vi "Toggle Lift Ears.vi"(8 "Delay":dbl, 9 "Distance Threshold":dbl, 10 "Avg Distance":dbl, 11 "Robot Mode":T1=enum."Teleop Enabled") -> (3 "Lift Output":bool)   [LabVIEW 2013]
uses:
  <vilib>/Rock Robotics/WPI/DriverStation/WPI_DriverStationRobotMode2.ctl
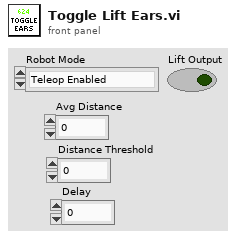
[diagram p1: front panel]
types:
  T1 = typedef "WPI_DriverStationRobotMode2.ctl" = enum16{"Autonomous Disabled", "Autonomous Enabled", "Teleop Disabled", "Teleop Enabled", "Timeout", "Finish", "Test Disabled", "Test Enabled"}
  T2 = enum16{"Wait for Auton", "Wait for Encoders", "On"}
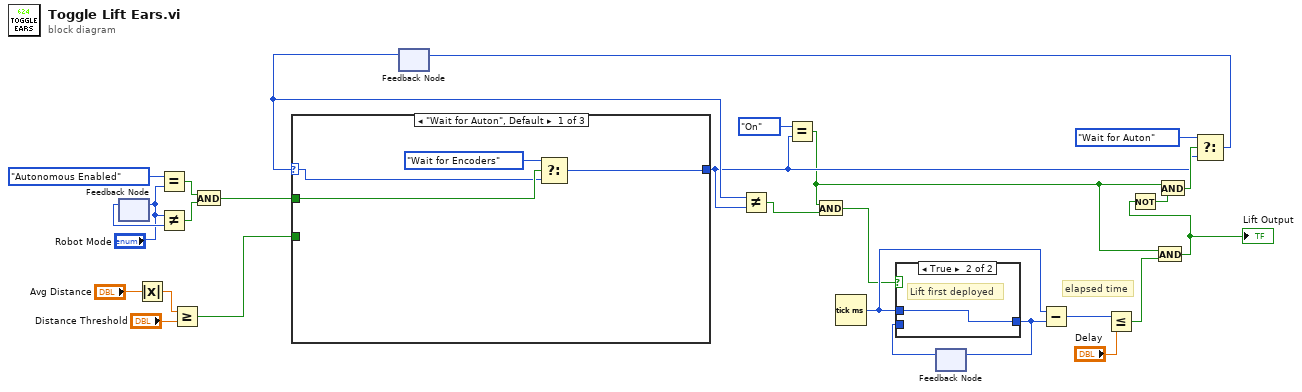
[diagram p0: block diagram]
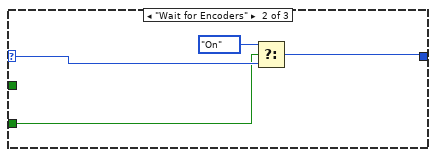
[diagram p3: hidden frame]
diagram:
  # "elapsed time"
  n1 = feedback #1() -> (w24:T1)  [unwired: 1 in]
  n2 = feedback-in #1("Robot Mode") -> ()
  n3 = Absolute Value(x="Avg Distance") -> (abs(x)=w17:dbl)
  n4 = Equal?(x=WPI_DriverStationRobotMode2."Autonomous Enabled", y="Robot Mode") -> (x = y?=w26:bool)
  n5 = Not Equal?(x="Robot Mode", y=w24) -> (x != y?=w27:bool)
  n6 = Greater Or Equal?(x=w17, y="Distance Threshold") -> (x >= y?=w21:bool)
  n7 = And(x=w26, y=w27) -> (x .and. y?=w22:bool)
  n8 = feedback #2() -> (w7:T2)  [unwired: 1 in]
  n9 = case shown="\"Wait for Auton\", Default" w7 {
    selector: w7 -> [w30 w34 w36]
    tunnel: w22 -> [w31 _ _]
    tunnel: [w28 w33 w36] -> w6
    tunnel: w21 -> [_ w32 _]
    frame "Wait for Auton", Default {
      n10 = Select(t=T2."Wait for Encoders", s=w31, f=w30) -> (s? t:f=w28:T2)
    }
    frame "Wait for Encoders" {
      n11 = Select(t=T2."On", s=w32, f=w34) -> (s? t:f=w33:T2)
    }
    frame "On" {
    }
  }
  n12 = Not Equal?(x=w7, y=w6) -> (x != y?=w5:bool)
  n13 = Equal?(x=T2."On" ("y"), y=w6) -> (x = y?=w3:bool)
  n14 = And(x=w3, y=w5) -> (x .and. y?=w4:bool)
  n15 = Tick Count (ms)() -> (millisecond timer value=w12:u32)
  n16 = feedback #3() -> (w14:u32)  [unwired: 1 in]
  n17 = case shown="True" w4 {
    tunnel: w14 -> [w37 _]
    tunnel: [w37 w38] -> w13
    tunnel: w12 -> [_ w38]
    frame False {
    }
    frame True {
      # "Lift first deployed"
    }
  }
  n18 = feedback-in #3(w13) -> ()
  n19 = Subtract(x=w12, y=w13) -> (x-y=w15:u32)
  n20 = Less Or Equal?(x=w15, y="Delay") -> (x <= y?=w2:bool)
  n21 = And(x=w3, y=w2) -> (x .and. y?=w1:bool)
  "Lift Output" <- w1
  n22 = Not(x=w1) -> (.not. x?=w10:bool)
  n23 = And(x=w3, y=w10) -> (x .and. y?=w9:bool)
  n24 = Select(t=T2."Wait for Auton", s=w9, f=w6) -> (s? t:f=w8:T2)
  n25 = feedback-in #2(w8) -> ()
